vi "Struct Close.vi"(7 "Typedef struct? (F)":bool, 10 "Typedef name":string, 11 "String in":string) -> (3 "String out":string)   [LabVIEW 2014, in "C Header Generator.lvlib"]
uses:
  C Header Generator.lvlib
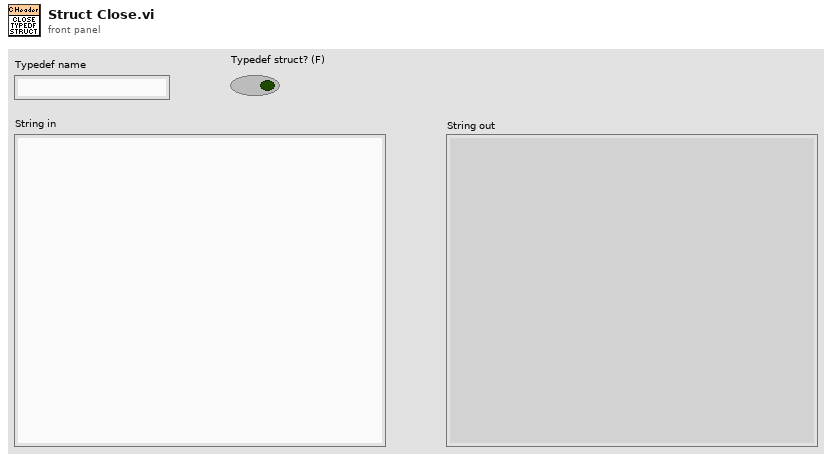
[diagram p1: front panel]
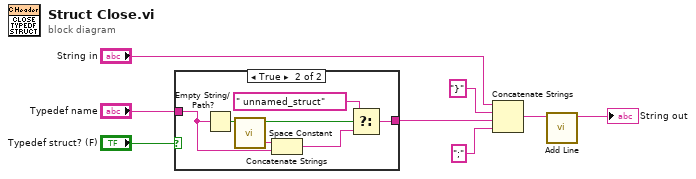
[diagram p0: block diagram]
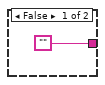
[diagram p2: hidden frame]
diagram:
  n1 = case shown="True" "Typedef struct? (F)" {
    tunnel: ["" w14] -> w3
    tunnel: "Typedef name" -> [_ w12]
    frame False {
    }
    frame True {
      n2 = Empty String/Path?(string/path=w12) -> (empty?=w15:bool)
      n3 = call <vilib>:"Space Constant.vi"() -> ("String"=w13:string)
      n4 = Concatenate Strings(w13, w12) -> (w11:string)
      n5 = Select(t=" unnamed_struct" ("string"), s=w15, f=w11) -> (s? t:f=w14:string)
    }
  }
  n6 = Concatenate Strings("String in", "}" ("string"), w3, ";" ("string")) -> (w5:string)
  n7 = call "Add Line.vi"("String in"=w5) -> ("String out"=→"String out":string)  [unwired: 10 in]
